vi "Configure Unbundle.vi"(8 "error in (no error)":errorcluster, 11 "Getter Generator in":refnum<class "Getter Generator.lvclass">) -> (0 "error out":errorcluster, 3 "Getter Generator out":refnum<class "Getter Generator.lvclass">)   [LabVIEW 2020, in "Method Generation.lvlib" / "Getter Generator.lvclass"]
uses:
  Getter Generator.lvclass
  <vilib>/Utility/traverseref.llb/TRef TravTarget.ctl
  Getter Generator.lvclass/Getter Generator.ctl
  <vilib>/Utility/traverseref.llb/VI Scripting - Traverse.lvlib
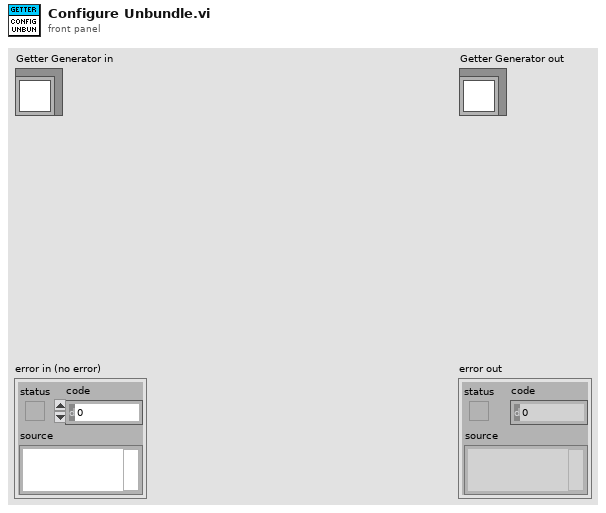
[diagram p1: front panel]
types:
  T1 = typedef "TRef TravTarget.ctl" = enum16{"FP", "BD", "Other"}
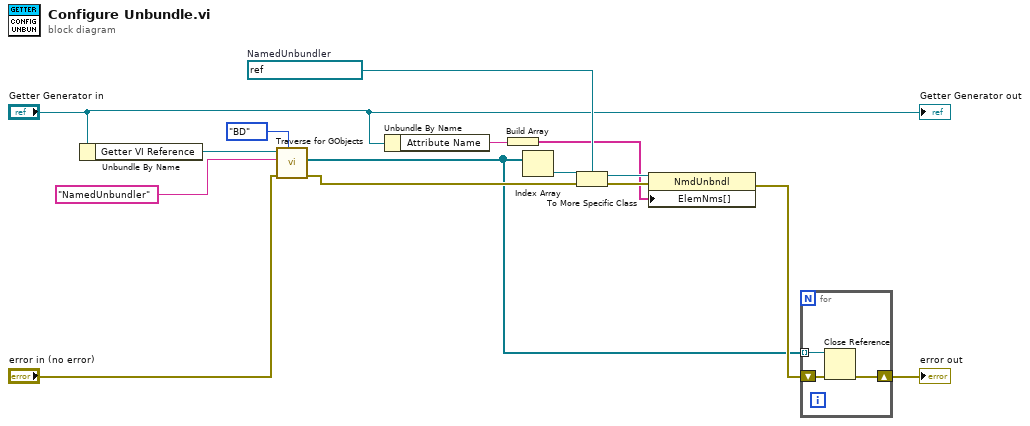
[diagram p0: block diagram]
diagram:
  w11 = refnum<vi> refnum  # NamedUnbundler
  n1 = Unbundle By Name("Getter Generator in") -> ("Getter VI Reference"=w15:refnum<vi>)
  n2 = call <vilib>:"Traverse for GObjects.vi"("Traverse Target"=TRef_TravTarget."BD", "error in (no error)"="error in (no error)", "Class Name"="NamedUnbundler", "VI Refnum"=w15) -> ("error out"=w12:errorcluster, "References"=w1:refnum<vi>[])  [unwired: 4 in, 2 out]
  n3 = Unbundle By Name("Getter Generator in") -> ("Attribute Name"=w4:string)
  n4 = Build Array(w4) -> (w3:string[])
  n5 = Index Array(array=w1) -> (element=w13:refnum<vi>)  [unwired: 1 in]
  n6 = To More Specific Class(target class=w11, reference=w13, error in=w12) -> (specific class reference=w9:refnum<vi>, error out=w8:errorcluster)
  n7 = property class="NmdUnbndl"(reference=w9, error in=w8, "ElemNms[]"=w3) -> (error out=w7:errorcluster)  [unwired: 1 out]
  n8 = for {
    shift-right: [w17] -> w2
    shift-left: w7 -> [w18]
    tunnel: w1 -> [w16] mode=indexing
    n9 = Close Reference(reference=w16, error in (no error)=w18) -> (error out=w17:errorcluster)
  }
  "error out" <- w2
  "Getter Generator out" <- "Getter Generator in"
